vi "Apply Speed.vi"(8 "error in (no error)":errorcluster, 11 "Tool Path in":refnum<class "Tool Path.lvclass">) -> (0 "error out":errorcluster, 3 "Tool Path out":refnum<class "Tool Path.lvclass">)   [LabVIEW 2019, in "Tool Path.lvclass"]
uses:
  Tool Path.lvclass
  Settings/ObjectSettings/ObjectSettings.lvclass/ObjectSettings.ctl
  Settings/Path Settings/Path Settings.lvclass
  C:/Users/Albro/Documents/GitHub/AFM-Lithography/lvsrc/Classes/Settings/ObjectSettings/ObjectSettings.lvclass
  Settings/ObjectSettings/ObjectSettings.lvclass
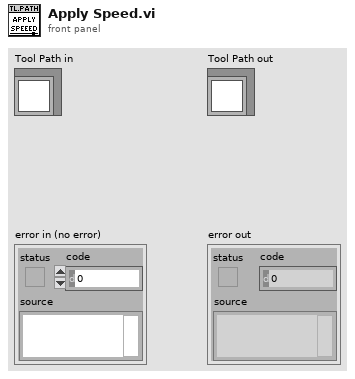
[diagram p1: front panel]
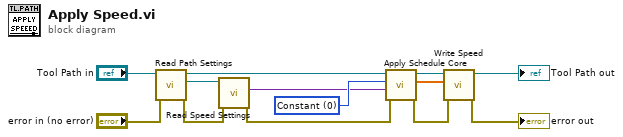
[diagram p0: block diagram]
diagram:
  w9 = u16 0 items=["Constant", "Ramp", "Function", "Formula"] ("Schedule")
  n1 = call-dynamic "Read Path Settings.vi"("error in (no error)"="error in (no error)", "Tool Path in"="Tool Path in") -> ("error out"=w12:errorcluster, "Path Settings.lvclass"=w13:refnum<class "Path Settings.lvclass">, "Tool Path out"=w8:refnum<class "Tool Path.lvclass">)  [unwired: 7 in]
  n2 = call "Read Speed Settings.vi"("error in (no error)"=w12, "ObjectSettings in"=w13) -> ("error out"=w2:errorcluster, "Settings"=w6:variant)  [unwired: 7 in, 1 out]
  n3 = call-dynamic "Apply Schedule Core.vi"("error in (no error)"=w2, "Settings"=w6, "Schedule"=w9, "Tool Object in"=w8) -> ("error out"=w3:errorcluster, "Schedule Array"=w1:dbl[], "Tool Object out"=w7:refnum<class "Tool Path.lvclass">)  [unwired: 5 in]
  n4 = call-dynamic "Write Speed.vi"("error in (no error)"=w3, "Speed"=w1, "Tool Object in"=w7) -> ("error out"=→"error out":errorcluster, "Tool Object out"=→"Tool Path out":refnum<class "Tool Path.lvclass">)  [unwired: 7 in]
